vi "Ch_data_title_pattern 16 (SubVI).vi"(8 "error in":errorcluster, 9 "Единица измерений":string) -> (0 "error out":errorcluster, 2 "Path":path, 3 "Byte Stream File out":refnum<file>)   [LabVIEW 2013]
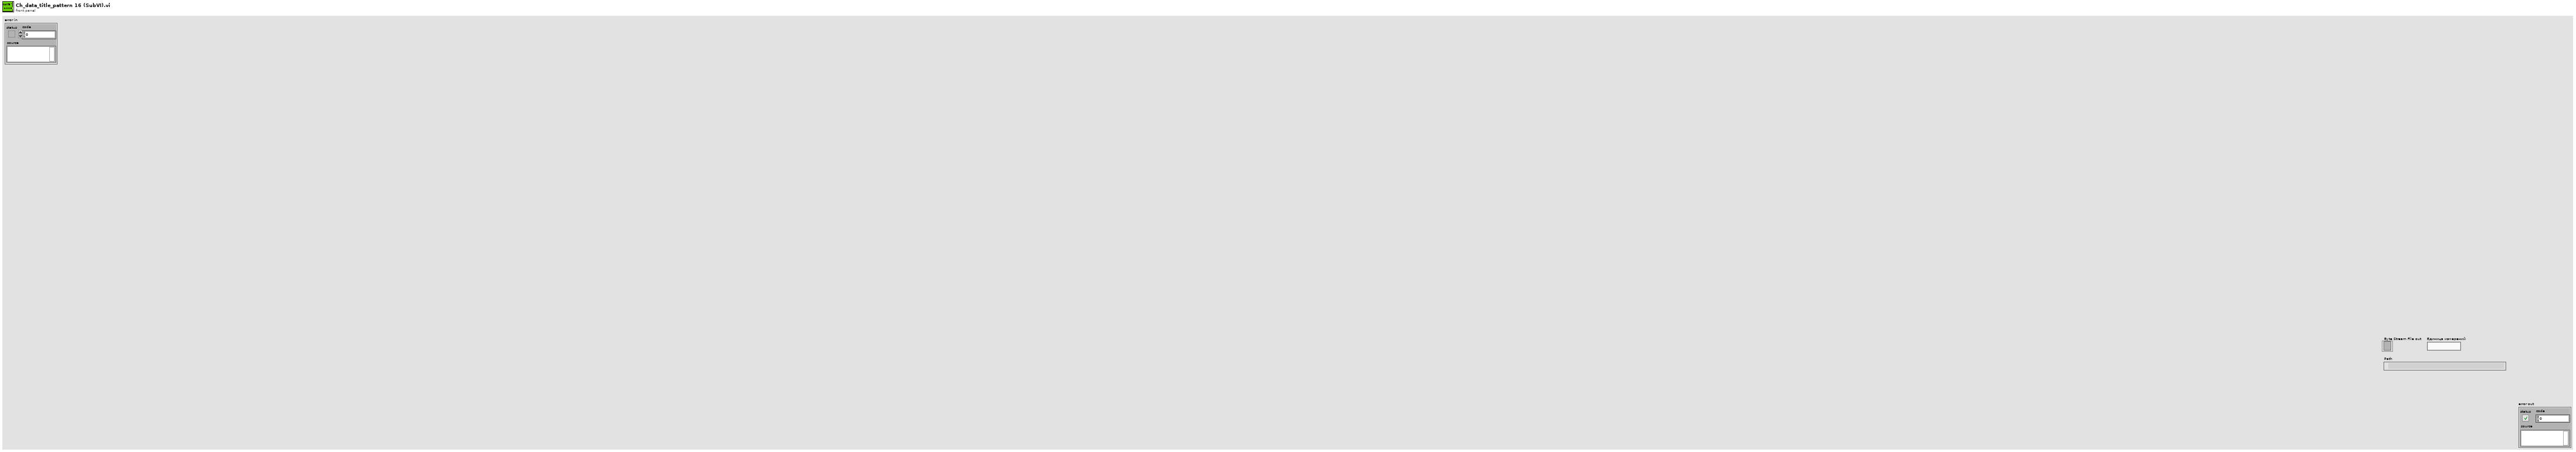
[diagram p1: front panel]
types:
  T1 = enum16{"open", "replace", "create", "open or create", "replace or create", "replace or create with confirmation"}
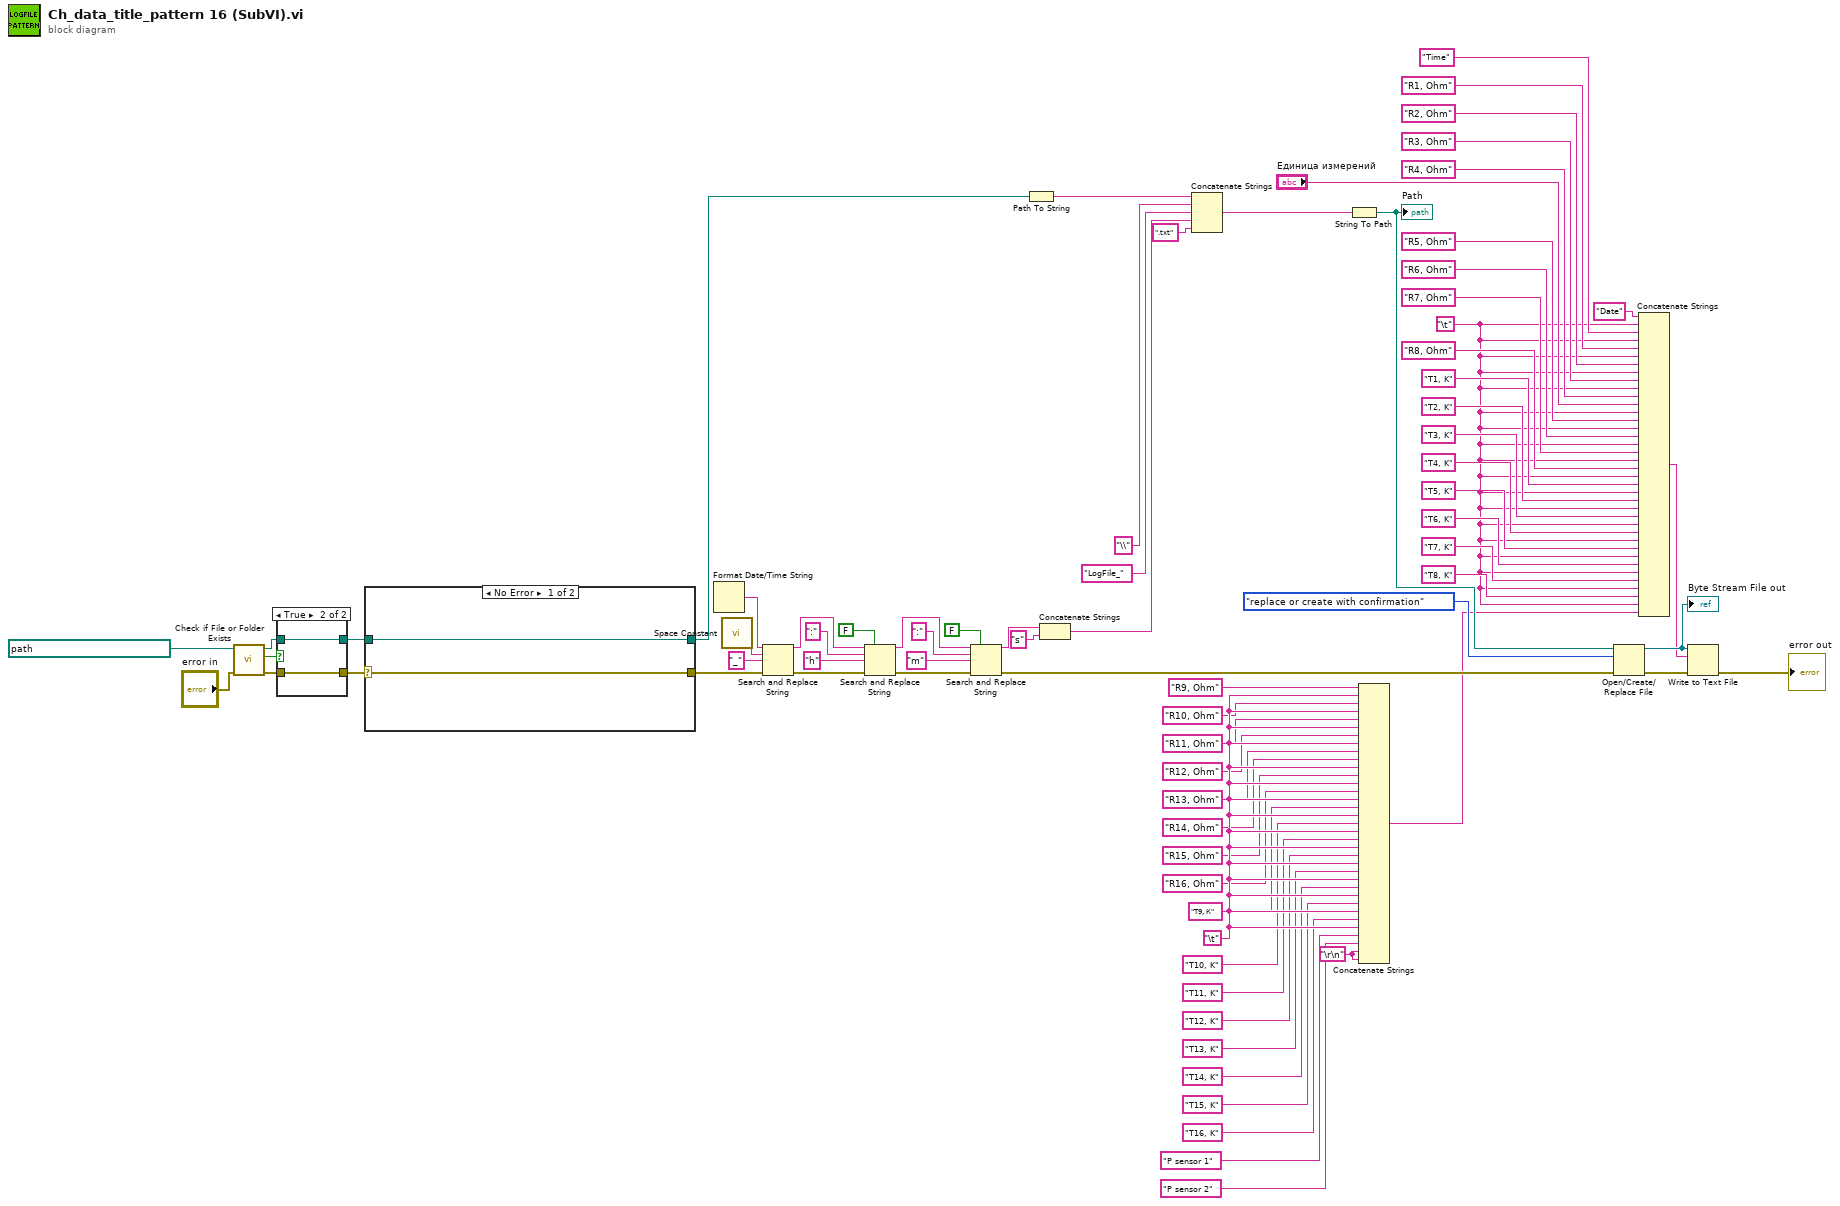
[diagram p0: block diagram]
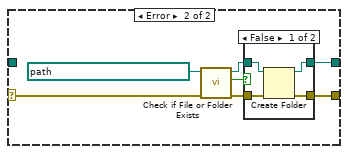
[diagram p2: hidden frame]
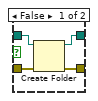
[diagram p4: hidden frame]
diagram:
  w21 = "\t"
  w22 = "\t"
  w3 = "\r\n"
  n1 = call <vilib>:"Check if File or Folder Exists.vi"("error in (no error)"="error in", "path"=path "D:/Лог-файл термометрии" ("path (use dialog)")) -> ("error out"=w65:errorcluster, "file or folder exists?"=w63:bool, "dup path"=w66:path)  [unwired: 7 out]
  n2 = case shown="True" w63 {
    tunnel: [w82 w84] -> w61
    tunnel: w66 -> [w81 w84]
    tunnel: w65 -> [w80 w83]
    tunnel: [w79 w83] -> w62
    frame False {
      n3 = Create Folder(path (use dialog)=w81, error in=w80) -> (created path=w82:path, error out=w79:errorcluster)  [unwired: 2 out]
    }
    frame True {
    }
  }
  n4 = case shown="No Error" w62 {
    selector: w62 -> [w85 w87]
    tunnel: w61 -> [w86 _]
    tunnel: [w86 w90] -> w37
    tunnel: [w85 w89] -> w38
    frame No Error {
    }
    frame Error {
      n5 = call <vilib>:"Check if File or Folder Exists.vi"("error in (no error)"=w87, "path"=path "C:/Лог-файл термометрии" ("path (use dialog)")) -> ("error out"=w92:errorcluster, "file or folder exists?"=w91:bool, "dup path"=w93:path)  [unwired: 7 out]
      n6 = case shown="False" w91 {
        tunnel: [w97 w99] -> w90
        tunnel: w93 -> [w96 w99]
        tunnel: w92 -> [w95 w98]
        tunnel: [w94 w98] -> w89
        frame False {
          n7 = Create Folder(path (use dialog)=w96, error in=w95) -> (created path=w97:path, error out=w94:errorcluster)  [unwired: 2 out]
        }
        frame True {
        }
      }
    }
  }
  n8 = Format Date/Time String() -> (date/time string=w59:string)  [unwired: 3 out]
  n9 = call <vilib>:"Space Constant.vi"() -> ("String"=w40:string)
  n10 = Search and Replace String(input string=w59, search string=w40, replace string="_" ("replace string (\"\")"), error in=w38) -> (result string=w42:string, error out=w52:errorcluster)  [unwired: 6 out]
  n11 = Search and Replace String(replace all?=FALSE ("replace all? (F)"), input string=w42, search string=":", replace string="h" ("replace string (\"\")"), error in=w52) -> (result string=w49:string, error out=w53:errorcluster)  [unwired: 5 out]
  n12 = Search and Replace String(replace all?=FALSE ("replace all? (F)"), input string=w49, search string=":", replace string="m" ("replace string (\"\")"), error in=w53) -> (result string=w54:string, error out=w36:errorcluster)  [unwired: 5 out]
  n13 = Path To String(path=w37) -> (string=w50:string)
  n14 = Concatenate Strings(w54, "s" ("string")) -> (w57:string)
  n15 = Concatenate Strings(w50, "\\" ("string"), "LogFile_" ("string"), w57, ".txt" ("default name")) -> (w39:string)
  n16 = String To Path(string=w39) -> (path=w35:path)
  "Path" <- w35
  n17 = Concatenate Strings("R9, Ohm" ("string"), w21, "R10, Ohm" ("string"), w21, "R11, Ohm" ("string"), w21, "R12, Ohm" ("string"), w21, "R13, Ohm" ("string"), "R14, Ohm" ("string"), w21, "R15, Ohm" ("string"), w21, "R16, Ohm" ("string"), w21, "T9, К" ("string"), w21, "T10, K" ("string"), w21, "T11, K" ("string"), w21, "T12, K" ("string"), w21, "T13, K" ("string"), w21, "T14, K" ("string"), w21, "T15, K" ("string"), w21, "T16, K" ("string"), w21, "P sensor 1" ("string"), "P sensor 2" ("string"), w3, w3) -> (w4:string)
  n18 = Open/Create/Replace File(file path (use dialog)=w35, error in=w36, operation (0:open)=T1."replace or create with confirmation") -> (refnum out=w72:refnum<file>, error out=w70:errorcluster)  [unwired: 4 out]
  "Byte Stream File out" <- w72
  n19 = Concatenate Strings("Date" ("string"), w22, "Time" ("string"), w22, "R1, Ohm" ("string"), w22, "R2, Ohm" ("string"), w22, "R3, Ohm" ("string"), w22, "R4, Ohm" ("string"), "Единица измерений", w22, "R5, Ohm" ("string"), w22, "R6, Ohm" ("string"), w22, "R7, Ohm" ("string"), w22, "R8, Ohm" ("string"), w22, "T1, K" ("string"), w22, "T2, K" ("string"), w22, "T3, K" ("string"), w22, "T4, K" ("string"), w22, "T5, K" ("string"), w22, "T6, K" ("string"), w22, "T7, K" ("string"), w22, "T8, K" ("string"), w22, w4) -> (w69:string)
  n20 = Write to Text File(file (use dialog)=w72, text=w69, error in=w70) -> (error out=→"error out":errorcluster)  [unwired: 3 out]
